vi "viserverUserAccess_addPrincipalToPrincipalArray.vi"(6 "PrivilegeID":u32, 7 "Access":u32(ring) items=["Grant", "Deny", "Unspecified"], 8 "error in (no error)":errorcluster, 9 "principal array in":T1[](array[typedef]) {"principal"."ID"."b7" format="%02x"; "principal"."ID"."b6" format="%02x"; "principal"."ID"."b5" format="%02x"; "principal"."ID"."b4" format="%02x"; "principal"."ID"."b3" format="%02x"; "principal"."ID"."b2" format="%02x"; "principal"."ID"."b1" format="%02x"; "principal"."ID"."b0" format="%02x"; "principal"."ID"."b15" format="%02x"; "principal"."ID"."b14" format="%02x"; "principal"."ID"."b13" format="%02x"; "principal"."ID"."b12" format="%02x"; "principal"."ID"."b11" format="%02x"; "principal"."ID"."b10" format="%02x"; "principal"."ID"."b9" format="%02x"; "principal"."ID"."b8" format="%02x"; "domain"."ID"."b7" format="%02x"; "domain"."ID"."b6" format="%02x"; "domain"."ID"."b5" format="%02x"; "domain"."ID"."b4" format="%02x"; "domain"."ID"."b3" format="%02x"; "domain"."ID"."b2" format="%02x"; "domain"."ID"."b1" format="%02x"; "domain"."ID"."b0" format="%02x"; "domain"."ID"."b15" format="%02x"; "domain"."ID"."b14" format="%02x"; "domain"."ID"."b13" format="%02x"; "domain"."ID"."b12" format="%02x"; "domain"."ID"."b11" format="%02x"; "domain"."ID"."b10" format="%02x"; "domain"."ID"."b9" format="%02x"; "domain"."ID"."b8" format="%02x"}, 10 "principal in":T1 {"principal"."ID"."b7" format="%02x"; "principal"."ID"."b6" format="%02x"; "principal"."ID"."b5" format="%02x"; "principal"."ID"."b4" format="%02x"; "principal"."ID"."b3" format="%02x"; "principal"."ID"."b2" format="%02x"; "principal"."ID"."b1" format="%02x"; "principal"."ID"."b0" format="%02x"; "principal"."ID"."b15" format="%02x"; "principal"."ID"."b14" format="%02x"; "principal"."ID"."b13" format="%02x"; "principal"."ID"."b12" format="%02x"; "principal"."ID"."b11" format="%02x"; "principal"."ID"."b10" format="%02x"; "principal"."ID"."b9" format="%02x"; "principal"."ID"."b8" format="%02x"; "domain"."ID"."b7" format="%02x"; "domain"."ID"."b6" format="%02x"; "domain"."ID"."b5" format="%02x"; "domain"."ID"."b4" format="%02x"; "domain"."ID"."b3" format="%02x"; "domain"."ID"."b2" format="%02x"; "domain"."ID"."b1" format="%02x"; "domain"."ID"."b0" format="%02x"; "domain"."ID"."b15" format="%02x"; "domain"."ID"."b14" format="%02x"; "domain"."ID"."b13" format="%02x"; "domain"."ID"."b12" format="%02x"; "domain"."ID"."b11" format="%02x"; "domain"."ID"."b10" format="%02x"; "domain"."ID"."b9" format="%02x"; "domain"."ID"."b8" format="%02x"}, 11 "ACL in":refnum<k20>) -> (0 "error out":errorcluster, 1 "principal array out":T1[](array[typedef]) {"principal"."ID"."b7" format="%02x"; "principal"."ID"."b6" format="%02x"; "principal"."ID"."b5" format="%02x"; "principal"."ID"."b4" format="%02x"; "principal"."ID"."b3" format="%02x"; "principal"."ID"."b2" format="%02x"; "principal"."ID"."b1" format="%02x"; "principal"."ID"."b0" format="%02x"; "principal"."ID"."b15" format="%02x"; "principal"."ID"."b14" format="%02x"; "principal"."ID"."b13" format="%02x"; "principal"."ID"."b12" format="%02x"; "principal"."ID"."b11" format="%02x"; "principal"."ID"."b10" format="%02x"; "principal"."ID"."b9" format="%02x"; "principal"."ID"."b8" format="%02x"; "domain"."ID"."b7" format="%02x"; "domain"."ID"."b6" format="%02x"; "domain"."ID"."b5" format="%02x"; "domain"."ID"."b4" format="%02x"; "domain"."ID"."b3" format="%02x"; "domain"."ID"."b2" format="%02x"; "domain"."ID"."b1" format="%02x"; "domain"."ID"."b0" format="%02x"; "domain"."ID"."b15" format="%02x"; "domain"."ID"."b14" format="%02x"; "domain"."ID"."b13" format="%02x"; "domain"."ID"."b12" format="%02x"; "domain"."ID"."b11" format="%02x"; "domain"."ID"."b10" format="%02x"; "domain"."ID"."b9" format="%02x"; "domain"."ID"."b8" format="%02x"}, 2 "added entry index":i32, 3 "ACL out":refnum<k20>)   [LabVIEW 2020]
doc: "Use this template to build a VI to use as a subVI."
uses:
  <vilib>/Platform/security/user/NI_Security Qualified Domain-Principal Pair.ctl
  <vilib>/Platform/security/user/NI_Security Domain.ctl
  <vilib>/Platform/security/user/NI_Security Identifier.ctl
  <vilib>/Platform/security/user/NI_Security Principal.ctl
  <vilib>/Platform/security/user/NI_Security PrincipalType.ctl
  <vilib>/Platform/security/user/NI_Security AccessRights_CloseRef.vi
  <vilib>/Platform/security/user/NI_Security ACE_CloseRef.vi
  <resource>/objmgr/Security.rc
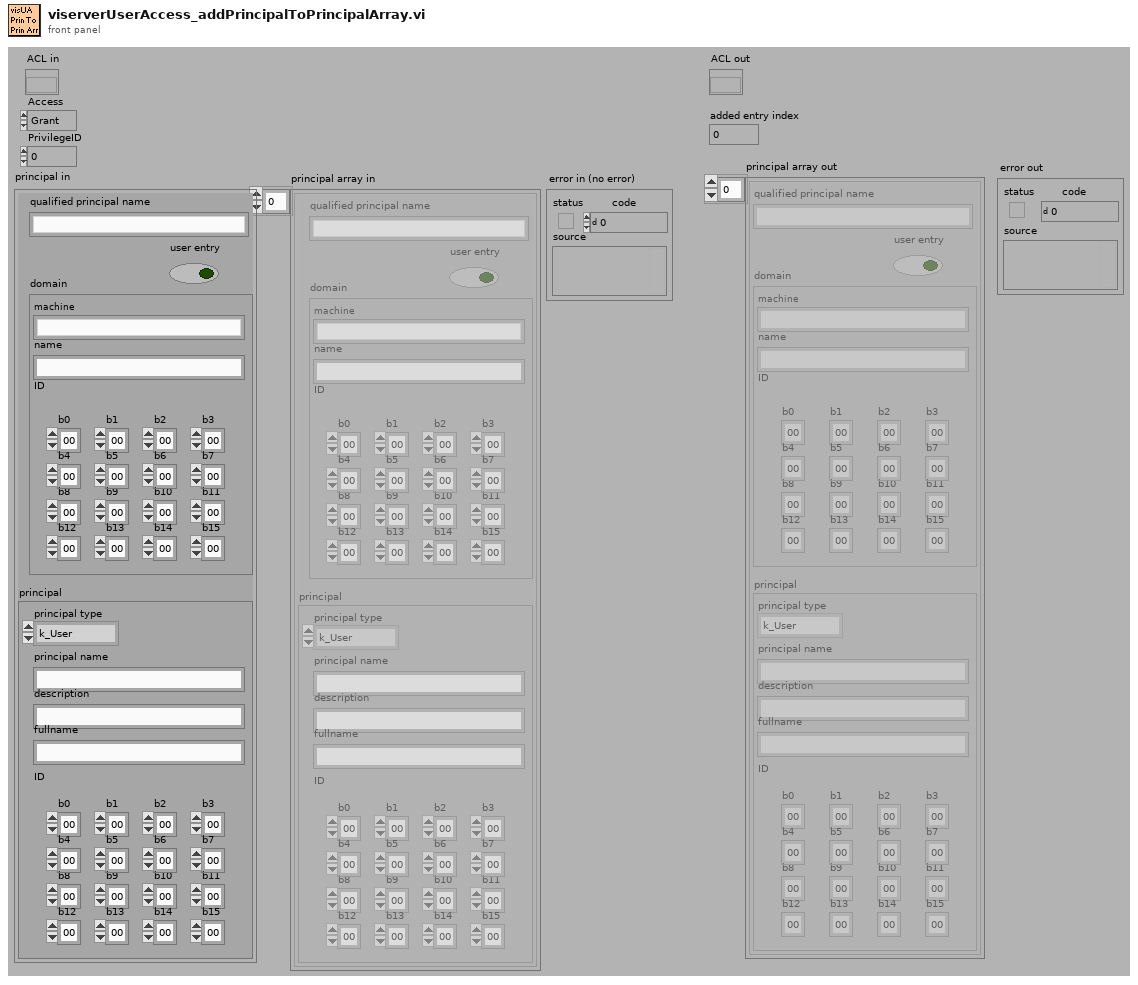
[diagram p1: front panel]
types:
  T1 = typedef "NI_Security Qualified Domain-Principal Pair.ctl" = cluster{"qualified principal name":string, "domain":T2, "principal":T4, "user entry":bool}
  T2 = typedef "NI_Security Domain.ctl" = cluster{"machine":string, "name":string, "ID":T3}
  T3 = typedef "NI_Security Identifier.ctl" = cluster{"b0":u8, "b1":u8, "b2":u8, "b3":u8, "b4":u8, "b5":u8, "b6":u8, "b7":u8, "b8":u8, "b9 ":u8, "b10":u8, "b11":u8, "b12":u8, "b13":u8, "b14":u8, "b15":u8}
  T4 = typedef "NI_Security Principal.ctl" = cluster{"principal type":T5, "principal name":string, "description":string, "fullname":string, "ID":T3}
  T5 = typedef "NI_Security PrincipalType.ctl" = enum16{"k_User", "k_Group"}
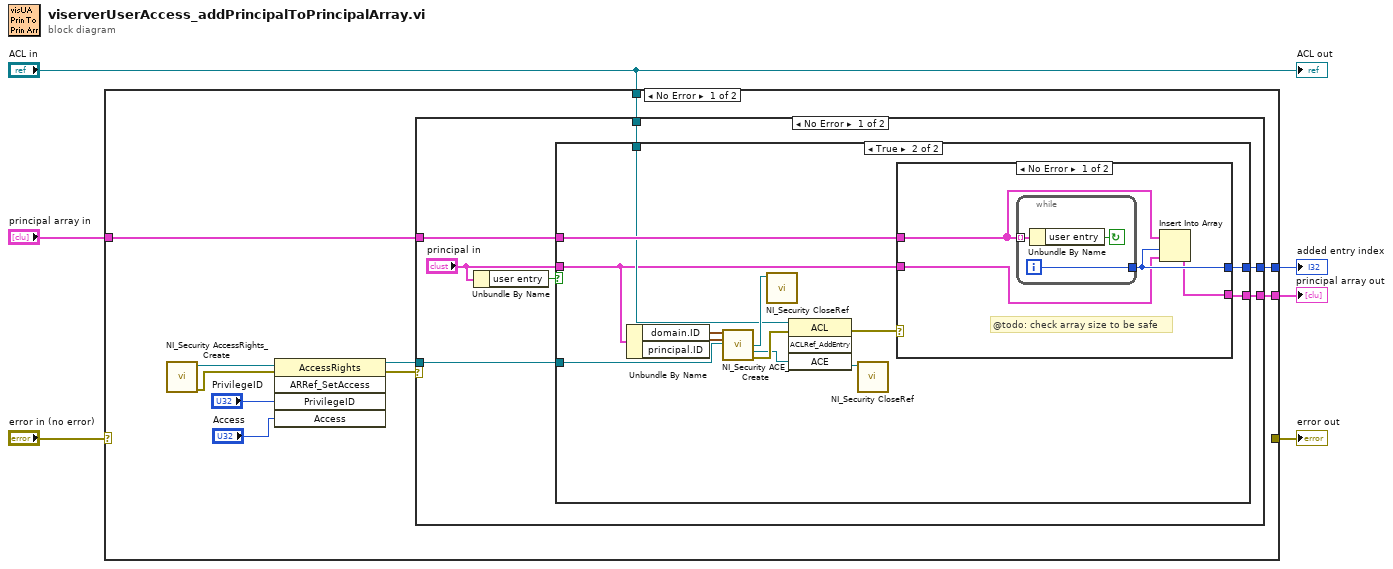
[diagram p0: block diagram]
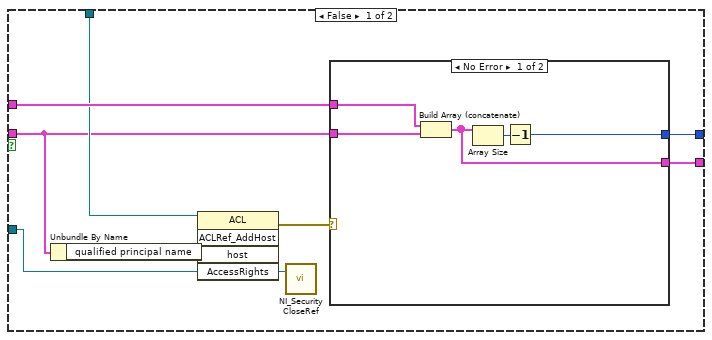
[diagram p2: hidden frame]
diagram:
  n1 = case shown="No Error" "error in (no error)" {
    selector: "error in (no error)" -> [_ w62]
    tunnel: [_ w62] -> w5
    tunnel: [w16 _] -> w4
    tunnel: "ACL in" -> [w13 _]
    tunnel: "principal array in" -> [w15 w61]
    tunnel: [w14 w61] -> w1
    frame No Error {
      n2 = call <vilib>:"NI_Security AccessRights_Create.vi"() -> ("error out"=w11:errorcluster, "AccessRights out"=w12:refnum<k20>)  [unwired: 10 in]
      n3 = invoke class="AccessRights" method="ARRef_SetAccess"(reference=w12, error in=w11, "PrivilegeID"="PrivilegeID", "Access"="Access") -> (reference out=w7:refnum<k20>, error out=w8:errorcluster)  [unwired: 1 in, 3 out]
      n4 = case shown="No Error" w8 {
        tunnel: [w23 _] -> w16
        tunnel: w15 -> [w22 w60]
        tunnel: [w21 w60] -> w14
        tunnel: w13 -> [w20 _]
        tunnel: w7 -> [w17 _]
        frame No Error {
          n5 = Unbundle By Name("principal in") -> ("user entry"=w18:bool)
          n6 = case shown="True" w18 {
            tunnel: [w29 w51] -> w23
            tunnel: w22 -> [w30 w50]
            tunnel: [w28 w49] -> w21
            tunnel: w20 -> [w27 w41]
            tunnel: "principal in" -> [w26 w40]
            tunnel: w17 -> [w24 w39]
            frame False {
              n7 = Unbundle By Name(w26) -> ("qualified principal name"=w25:string)
              n8 = invoke class="ACL" method="ACLRef_AddHost"(reference=w27, "host"=w25, "AccessRights"=w24) -> (error out=w31:errorcluster, "AccessRights"=w32:refnum<k20>)  [unwired: 2 in, 3 out]
              n9 = call-poly <vilib>:"NI_Security CloseRef.vi"("security refnum"=w32) -> ()  [unwired: 10 in, 1 out]
              n10 = case shown="No Error" w31 {
                tunnel: [w37 w38] -> w28
                tunnel: [w35 _] -> w29
                tunnel: w26 -> [w34 _]
                tunnel: w30 -> [w33 w38]
                frame No Error {
                  n11 = Build Array (concatenate)(w33, w34) -> (w37:T1[])
                  n12 = Array Size(array=w37) -> (size(s)=w36:i32)
                  n13 = Decrement(x=w36) -> (x-1=w35:i32)
                }
                frame Error {
                }
              }
            }
            frame True {
              n14 = Unbundle By Name(w40) -> ("domain.ID"=w43:T3, "principal.ID"=w44:T3)
              n15 = call <vilib>:"NI_Security ACE_Create.vi"("DomainId in"=w43, "PrincipalID in"=w44, "AccessRights in"=w39) -> ("AccessRights out"=w47:refnum<k20>, "ACE"=w45:refnum<k20>, "error out"=w46:errorcluster)  [unwired: 8 in, 2 out]
              n16 = call-poly <vilib>:"NI_Security CloseRef.vi"("security refnum"=w47) -> ()  [unwired: 10 in, 1 out]
              n17 = invoke class="ACL" method="ACLRef_AddEntry"(reference=w41, error in=w46, "ACE"=w45) -> (error out=w42:errorcluster, "ACE"=w48:refnum<k20>)  [unwired: 1 in, 2 out]
              n18 = call-poly <vilib>:"NI_Security CloseRef.vi"("security refnum"=w48) -> ()  [unwired: 10 in, 1 out]
              n19 = case shown="No Error" w42 {
                tunnel: [w53 w59] -> w49
                tunnel: w50 -> [w55 w59]
                tunnel: [w54 _] -> w51
                tunnel: w40 -> [w52 _]
                frame No Error {
                  # "@todo: check array size to be safe"
                  n20 = while {
                    tunnel: w55 -> [w58] mode=indexing
                    tunnel: [w56] -> w54
                    i -> [w56]
                    stop <- w57 continue-if-true
                    n21 = Unbundle By Name(w58) -> ("user entry"=w57:bool)
                  }
                  n22 = Insert Into Array(array=w55, index=w54, new element=w52) -> (w53:T1[])
                }
                frame Error {
                  # "@todo: what index should be returned on error?"
                }
              }
            }
          }
        }
        frame Error {
        }
      }
    }
    frame Error {
    }
  }
  "error out" <- w5
  "added entry index" <- w4
  "principal array out" <- w1
  "ACL out" <- "ACL in"
